vi "2020-PulleyMotor.vi"(8 "error in":errorcluster, 11 "Boolean":bool) -> (0 "error out":errorcluster, 3 "Pulley Stator Current":dbl)   [LabVIEW 2019]
uses:
  2020LabView/Robot Global Data.vi
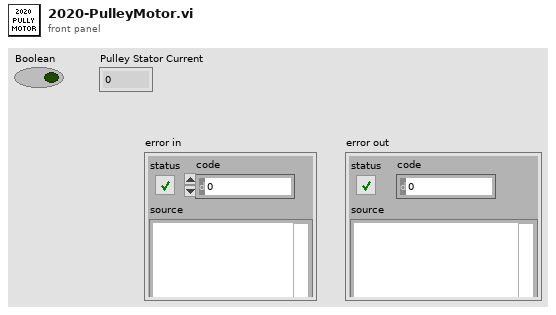
[diagram p1: front panel]
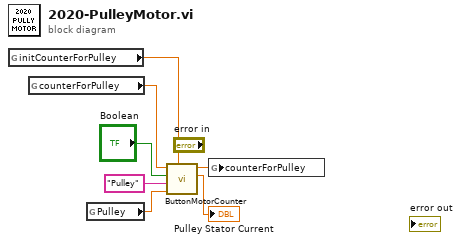
[diagram p0: block diagram]
diagram:
  n1 = global read "Robot Global Data.vi" "initCounterForPulley"() -> (w6:dbl)
  n2 = global read "Robot Global Data.vi" "counterForPulley"() -> (w2:dbl)
  n3 = global read "Robot Global Data.vi" "Pulley"() -> (w5:dbl)
  n4 = call "ButtonMotorCounter.vi"("counterStartValue"=w6, "Motor Set Point"=w5, "refnum name"="Pulley", "Boolean"="Boolean", "counterForIntake in"=w2) -> ("Stator Current"=→"Pulley Stator Current":dbl, "counterForIntake out"=w3:dbl)  [unwired: 5 in]
  n5 = global write "Robot Global Data.vi" "counterForPulley"(w3) -> ()
